vi "add to memory format.vi"(8 "error in":errorcluster, 9 "NISE_CEF_serializable configuration in":refnum<class "NISE_CEF_serializable configuration.lvclass">, 10 "parent ID":string, 11 "memory hierarchy in":T1) -> (0 "error out":errorcluster, 3 "memory hierarchy out":T1)   [LabVIEW 2013, in "NISE_CEF_TreeSerializer.lvlib"]
uses:
  NISE_CEF_TreeSerializer.lvlib
  memory hierarchy.ctl
  hierarchy element.ctl
  serializable configuration/NISE_CEF_serializable configuration.lvclass
  serializable configuration/NISE_CEF_serializable configuration.lvclass/NISE_CEF_serializable configuration.ctl
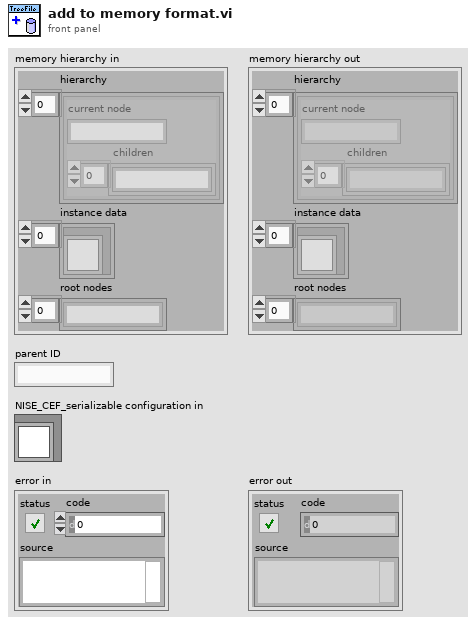
[diagram p1: front panel]
types:
  T1 = typedef "NISE_CEF_TreeSerializer.lvlib/memory hierarchy.ctl" = cluster{"hierarchy":T2[], "instance data":refnum<class "NISE_CEF_serializable configuration.lvclass">[], "root nodes":string[]}
  T2 = typedef "NISE_CEF_TreeSerializer.lvlib/hierarchy element.ctl" = cluster{"current node":string, "children":string[]}
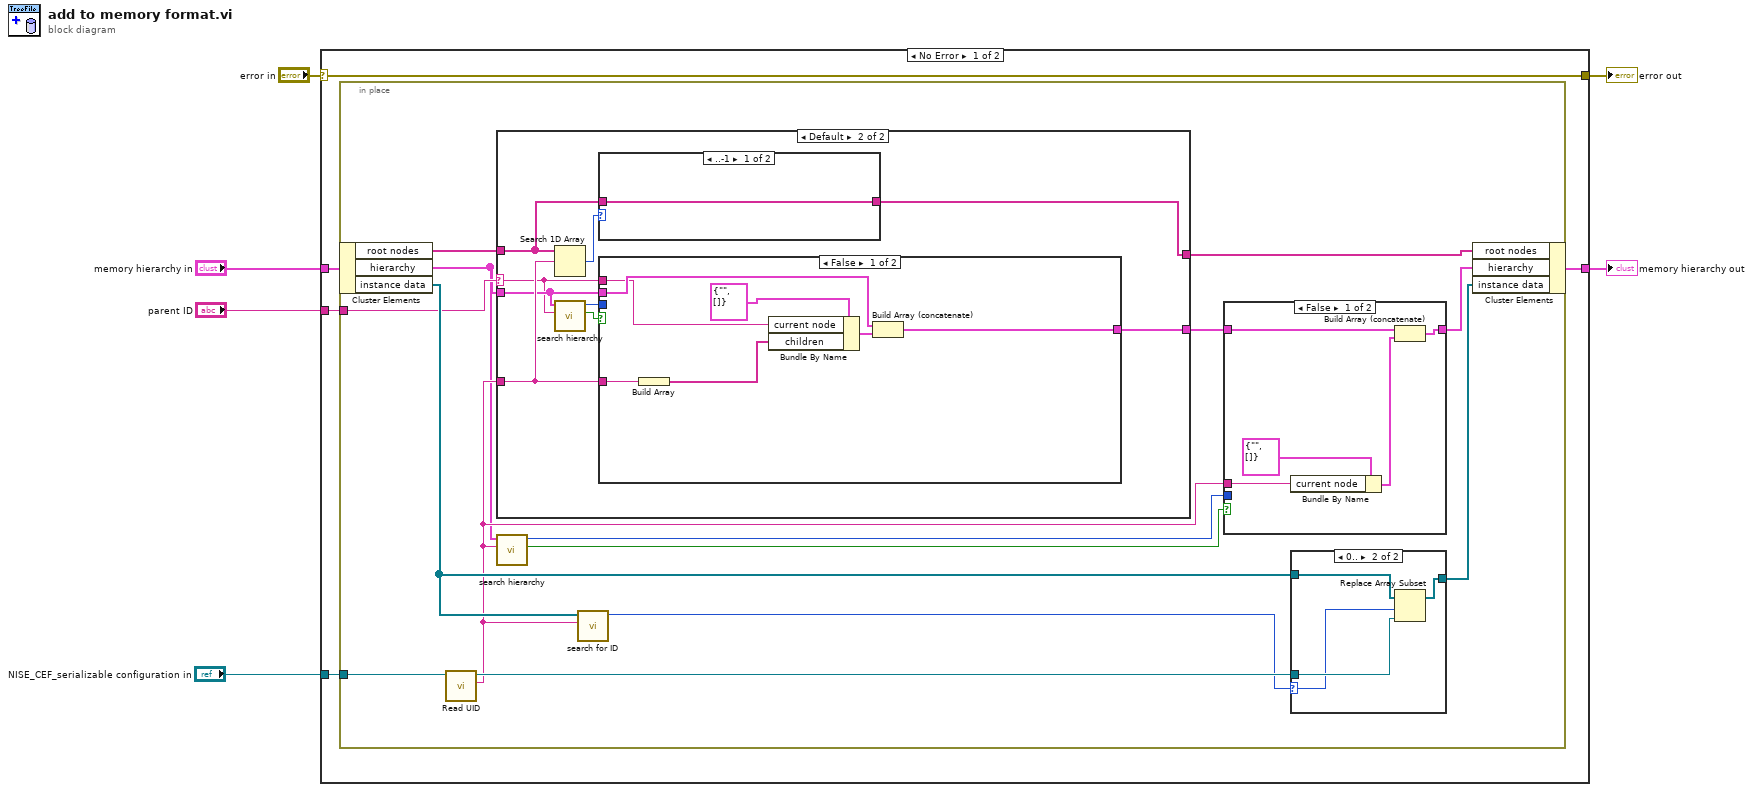
[diagram p0: block diagram]
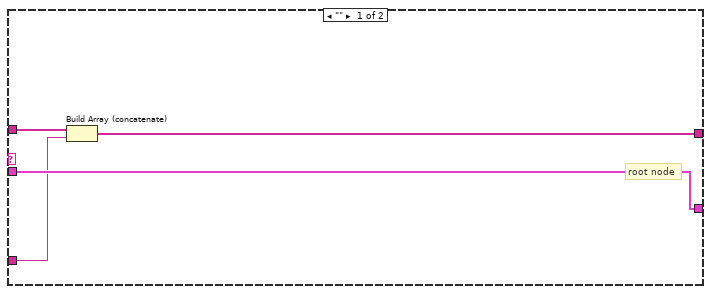
[diagram p2: hidden frame]
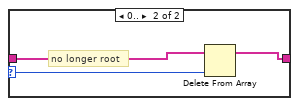
[diagram p3: hidden frame]
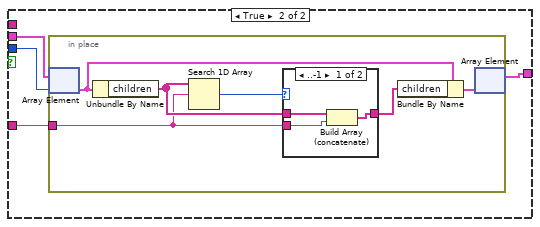
[diagram p4: hidden frame]
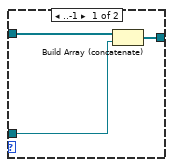
[diagram p7: hidden frame]
diagram:
  n1 = case shown="No Error" "error in" {
    selector: "error in" -> [w7 w78]
    tunnel: [w11 w77] -> w6
    tunnel: "memory hierarchy in" -> [w10 w77]
    tunnel: "parent ID" -> [w9 _]
    tunnel: "NISE_CEF_serializable configuration in" -> [w8 _]
    tunnel: [w7 w78] -> w1
    frame No Error {
      n2 = in-place {
        in-place-border: w8 -> [w25]
        in-place-border: w9 -> [w19]
        n3 = in-place-cluster #1(w10) -> ("root nodes"=w18:string[], "hierarchy"=w13:T2[], "instance data"=w23:refnum<class "NISE_CEF_serializable configuration.lvclass">[])
        n4 = call "Read UID.vi"("configuration in"=w25) -> ("instance id"=w14:string, "configuration out"=w22:refnum<class "NISE_CEF_serializable configuration.lvclass">)  [unwired: 8 in, 1 out]
        n5 = case shown="Default" w19 {
          selector: w19 -> [_ w30]
          tunnel: w13 -> [w29 w31]
          tunnel: [w29 w36] -> w21
          tunnel: w14 -> [w26 w35]
          tunnel: w18 -> [w28 w33]
          tunnel: [w27 w32] -> w17
          frame "" {
            # "root node"
            n6 = Build Array (concatenate)(w28, w26) -> (w27:string[])
          }
          frame Default {
            n7 = Search 1D Array(1D array=w33, element=w35) -> (index of element=w34:i32)  [unwired: 1 in]
            n8 = call "search hierarchy.vi"("ID"=w30, "hierarchy"=w31) -> ("found"=w38:bool, "index"=w37:i32)  [unwired: 8 in]
            n9 = case shown="..-1" w34 {
              selector: w34 -> [_ w41]
              tunnel: w33 -> [w39 w42]
              tunnel: [w39 w40] -> w32
              frame ..-1 {
              }
              frame 0.. {
                # "no longer root"
                n10 = Delete From Array(array=w42, index=w41) -> (array with subset deleted=w40:string[])  [unwired: 1 in, 1 out]
              }
            }
            n11 = case shown="False" w38 {
              tunnel: w31 -> [w47 w53]
              tunnel: w37 -> [_ w52]
              tunnel: [w44 w51] -> w36
              tunnel: w35 -> [w46 w50]
              tunnel: w30 -> [w43 _]
              frame False {
                n12 = Build Array(w46) -> (w45:string[])
                n13 = Bundle By Name(cluster=T2 {"current node"="", "children"=[]} ("hierarchy"), "current node"=w43, "children"=w45) -> (w49:T2)
                n14 = Build Array (concatenate)(w47, w49) -> (w44:T2[])
              }
              frame True {
                n15 = in-place {
                  in-place-border: w50 -> [w55]
                  n16 = in-place-array #2(w53, w52) -> (w59:T2)
                  n17 = Unbundle By Name(w59) -> ("children"=w56:string[])
                  n18 = Search 1D Array(1D array=w56, element=w55) -> (index of element=w57:i32)  [unwired: 1 in]
                  n19 = case shown="..-1" w57 {
                    tunnel: w56 -> [w62 w63]
                    tunnel: w55 -> [w61 _]
                    tunnel: [w60 w63] -> w54
                    frame ..-1 {
                      n20 = Build Array (concatenate)(w62, w61) -> (w60:string[])
                    }
                    frame 0.. {
                    }
                  }
                  n21 = Bundle By Name(cluster=w59, "children"=w54) -> (w58:T2)
                  n22 = in-place-array #2(w58) -> (w51:T2[])  [unwired: 1 out]
                }
              }
            }
          }
        }
        n23 = call "search hierarchy.vi"("ID"=w14, "hierarchy"=w13) -> ("found"=w15:bool, "index"=w16:i32)  [unwired: 8 in]
        n24 = call "search for ID.vi"("instance id"=w14, "instance data"=w23) -> ("index"=w12:i32)  [unwired: 9 in]
        n25 = case shown="False" w15 {
          tunnel: w16 -> [_ _]
          tunnel: w21 -> [w68 w69]
          tunnel: [w67 w69] -> w20
          tunnel: w14 -> [w65 _]
          frame False {
            n26 = Bundle By Name(cluster=T2 {"current node"="", "children"=[]} ("hierarchy"), "current node"=w65) -> (w64:T2)
            n27 = Build Array (concatenate)(w68, w64) -> (w67:T2[])
          }
          frame True {
          }
        }
        n28 = case shown="0.." w12 {
          selector: w12 -> [_ w73]
          tunnel: [w71 w75] -> w24
          tunnel: w23 -> [w70 w76]
          tunnel: w22 -> [w72 w74]
          frame ..-1 {
            n29 = Build Array (concatenate)(w70, w72) -> (w71:refnum<class "NISE_CEF_serializable configuration.lvclass">[])
          }
          frame 0.. {
            n30 = Replace Array Subset(array=w76, new element=w74, index=w73) -> (w75:refnum<class "NISE_CEF_serializable configuration.lvclass">[])
          }
        }
        n31 = in-place-cluster #1("root nodes"=w17, "hierarchy"=w20, "instance data"=w24) -> (w11:T1)
      }
    }
    frame Error {
    }
  }
  "memory hierarchy out" <- w6
  "error out" <- w1
